vi "Boolean to Data Type.vi"(8 "error in (no error)":errorcluster, 11 "Boolean":bool) -> (0 "error out":errorcluster, 3 "Boolean out":refnum<class "Boolean.lvclass">)   [LabVIEW 2019, in "Boolean.lvclass"]
uses:
  <vilib>/gpm_packages/@cs/data-type-serializer/source/Boolean/Boolean.lvclass
  <vilib>/gpm_packages/@cs/data-type-serializer/source/Boolean/Boolean.lvclass/Boolean.ctl
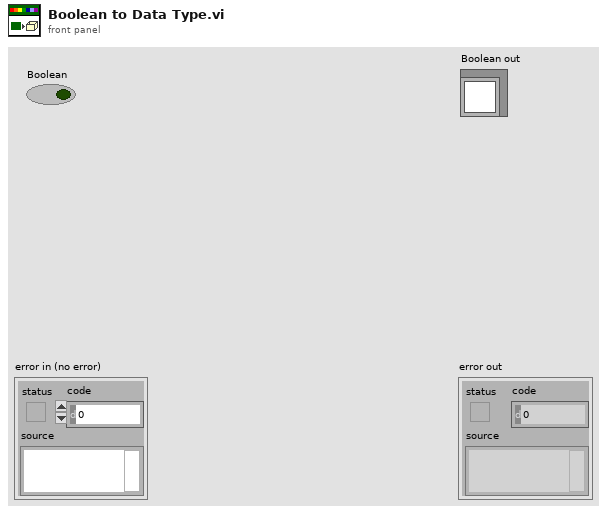
[diagram p1: front panel]
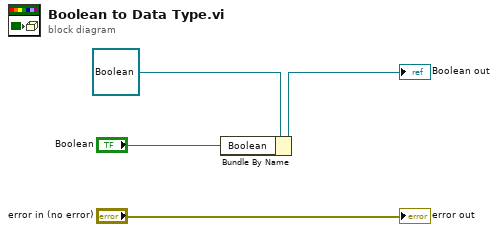
[diagram p0: block diagram]
diagram:
  n1 = Bundle By Name(cluster=refnum<class "Boolean.lvclass"> refnum ("Boolean in"), "Boolean"="Boolean") -> (→"Boolean out":refnum<class "Boolean.lvclass">)
  "error out" <- "error in (no error)"
